vi "GetContextHelpInfo.vi"(0 "reference":refnum<class "AbstractEdge.lvclass">, 1 "MousePos":T1 {"y" format="%.2f"; "x" format="%.2f"}, 5 "error in (no error)":errorcluster) -> (14 "reference out":refnum<class "AbstractEdge.lvclass">, 15 "ContextHelpInfoExist":bool, 16 "ContextHelpInfo":variant, 17 "Rows":string[](array[string]), 19 "error out":errorcluster)   [LabVIEW 2016, in "AbstractEdge.lvclass"]
doc: "GetContextHelpInfo"
uses:
  <resource>/Framework/Providers/Open_GDS/UML/AbstractEdge_class/AbstractEdge.lvclass
  <resource>/Framework/Providers/Open_GDS/UML/General/Point/Point Point2D.ctl
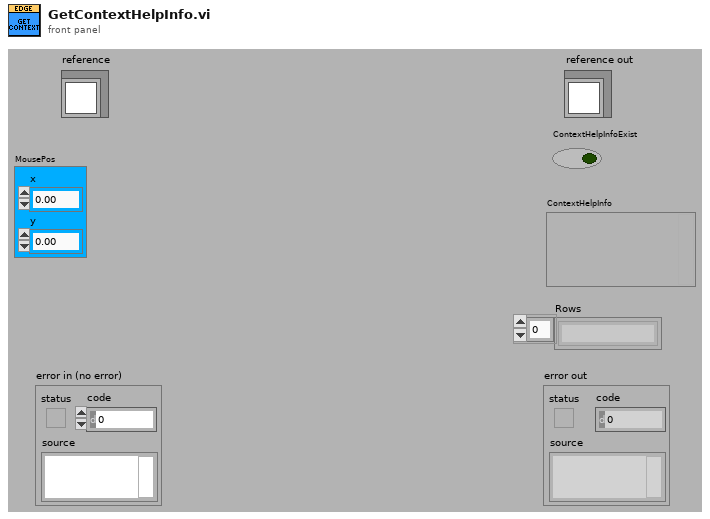
[diagram p1: front panel]
types:
  T1 = typedef "Point Point2D.ctl" = cluster{"x":dbl, "y":dbl}
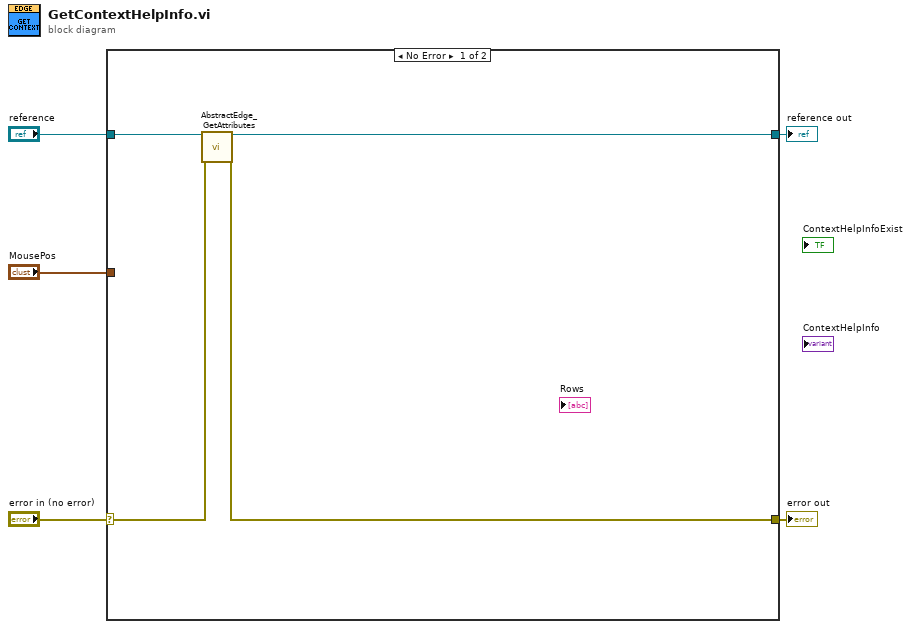
[diagram p0: block diagram]
diagram:
  n1 = case shown="No Error" "error in (no error)" {
    selector: "error in (no error)" -> [w6 w10]
    tunnel: "reference" -> [w9 w11]
    tunnel: [w8 w10] -> w4
    tunnel: [w7 w11] -> w3
    tunnel: "MousePos" -> [_ _]
    frame No Error {
      n2 = call <resource>:"AbstractEdge_GetAttributes.vi"("reference in"=w9, "error in (no error)"=w6) -> ("reference out"=w7:refnum<class "AbstractEdge.lvclass">, "error out"=w8:errorcluster)  [unwired: 1 in, 15 out]
    }
    frame Error {
    }
  }
  "reference out" <- w3
  "error out" <- w4
